vi "Day 9-2.vi"() -> ()   [LabVIEW 2020]
uses:
  Visit Item.ctl
panel:
  out "Answer":i32
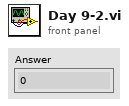
[diagram p1: front panel]
types:
  T1 = typedef "Visit Item.ctl" = cluster{"To":cluster{"Row":i32, "Col":i32}, "From":cluster{"Row":i32, "Col":i32}}
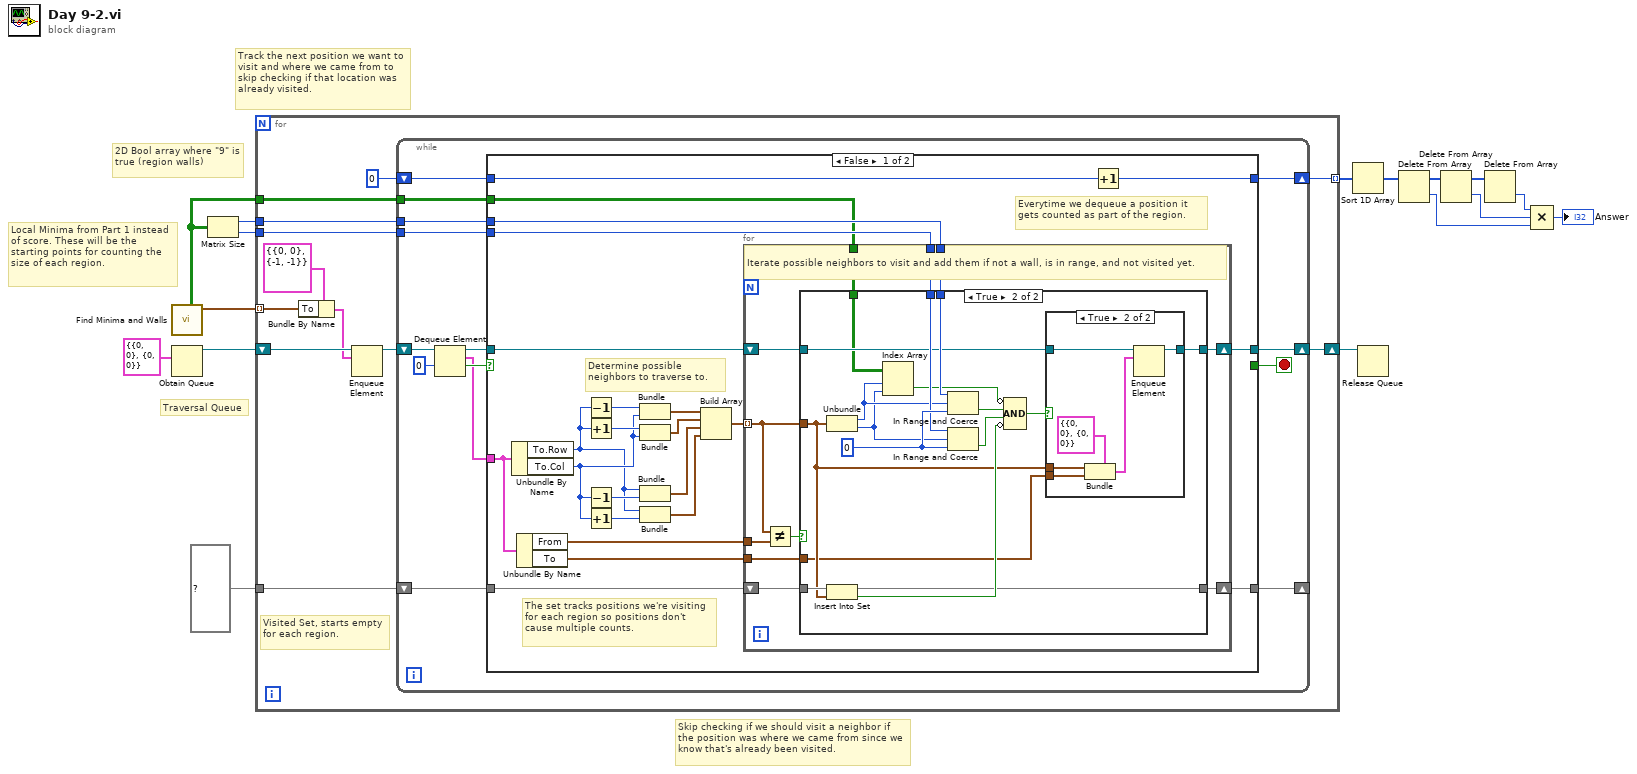
[diagram p0: block diagram]
diagram:
  # "Skip checking if we should visit a neighbor if the position was where we came from since we know that's already been visited."
  # "Track the next position we want to visit and where we came from to skip checking if that location was already visited."
  # "Local Minima from Part 1 instead of score. These will be the starting points for counting the size of each region."
  # "2D Bool array where \"9\" is true (region walls)"
  # "Traversal Queue"
  n1 = call "Find Minima and Walls.vi"() -> ("Low Points"=w16:cluster{i32, i32}[], "Wall"=w3:bool[][])  [unwired: 10 in]
  n2 = Obtain Queue(element data type=T1 {"To"={"Row"=0, "Col"=0}, "From"={"Row"=0, "Col"=0}} ("Visit Item")) -> (queue out=w14:refnum<queue>)  [unwired: 4 in, 2 out]
  n3 = Matrix Size(0:w3) -> (1:w2:i32, 2:w1:i32)
  n4 = for {
    tunnel: w16 -> [w27] mode=indexing
    shift-right: [w21] -> w12
    shift-left: w14 -> [w26]
    tunnel: w3 -> [w22]
    tunnel: set{cluster{"Row":i32, "Col":i32}} {} ("set") -> [w24]
    tunnel: [w19] -> w11 mode=indexing
    tunnel: w2 -> [w18]
    tunnel: w1 -> [w17]
    # "Visited Set, starts empty for each region."
    n5 = Bundle By Name(cluster=T1 {"To"={"Row"=0, "Col"=0}, "From"={"Row"=-1, "Col"=-1}} ("Visit Item"), "To"=w27) -> (w25:T1)
    n6 = Enqueue Element(queue=w26, element=w25) -> (queue out=w23:refnum<queue>)  [unwired: 2 in, 2 out]
    n7 = while {
      tunnel: w22 -> [w37]
      shift-right: [w31] -> _
      shift-left: w24 -> [w36]
      shift-right: [w34] -> w21
      shift-left: w23 -> [w42]
      shift-right: [w32] -> w19
      shift-left: 0 -> [w33]
      tunnel: w18 -> [w30]
      tunnel: w17 -> [w29]
      stop <- w35 stop-if-true
      n8 = Dequeue Element(queue=w42, timeout in ms (-1)=0) -> (queue out=w40:refnum<queue>, element=w38:T1, timed out?=w39:bool)  [unwired: 1 in, 1 out]
      n9 = case shown="False" w39 {
        selector: w39 -> [_ w106]
        tunnel: w40 -> [w52 w105]
        tunnel: w38 -> [w65 _]
        tunnel: w37 -> [w44 _]
        tunnel: w36 -> [w50 w103]
        tunnel: [_ w106] -> w35
        tunnel: [w51 w105] -> w34
        tunnel: w33 -> [w54 w104]
        tunnel: [w53 w104] -> w32
        tunnel: [w49 w103] -> w31
        tunnel: w30 -> [w47 _]
        tunnel: w29 -> [w46 _]
        frame False {
          # "The set tracks positions we're visiting for each region so positions don't cause multiple counts."
          # "Determine possible neighbors to traverse to."
          # "Everytime we dequeue a position it gets counted as part of the region."
          n10 = Unbundle By Name(w65) -> ("To.Row"=w59:i32, "To.Col"=w62:i32)
          n11 = Unbundle By Name(w65) -> ("From"=w45:cluster{"Row":i32, "Col":i32}, "To"=w43:cluster{"Row":i32, "Col":i32})
          n12 = Decrement(x=w59) -> (x-1=w64:i32)
          n13 = Increment(x=w59) -> (x+1=w63:i32)
          n14 = Decrement(x=w62) -> (x-1=w61:i32)
          n15 = Increment(x=w62) -> (x+1=w60:i32)
          n16 = Bundle(w64, "Col"=w62) -> (w58:cluster{i32, "Col":i32})  [unwired: 1 in]
          n17 = Bundle(w63, "Col"=w62) -> (w57:cluster{i32, "Col":i32})  [unwired: 1 in]
          n18 = Bundle("Row"=w59, w61) -> (w56:cluster{"Row":i32, i32})  [unwired: 1 in]
          n19 = Bundle("Row"=w59, w60) -> (w55:cluster{"Row":i32, i32})  [unwired: 1 in]
          n20 = Build Array(w58, w57, w56, w55) -> (w48:cluster{"Row":i32, "Col":i32}[])
          n21 = for {
            shift-right: [w67] -> w51
            shift-left: w52 -> [w70]
            shift-right: [w66] -> w49
            shift-left: w50 -> [w76]
            tunnel: w48 -> [w72] mode=indexing
            tunnel: w47 -> [w75]
            tunnel: w46 -> [w74]
            tunnel: w45 -> [w73]
            tunnel: w44 -> [w69]
            tunnel: w43 -> [w68]
            # "Iterate possible neighbors to visit and add them if not a wall, is in range, and not visited yet."
            n22 = Not Equal?(x=w72, y=w73) -> (x != y?=w71:bool)
            n23 = case shown="True" w71 {
              tunnel: w76 -> [w78 w95]
              tunnel: w75 -> [_ w93]
              tunnel: w74 -> [_ w92]
              tunnel: w72 -> [_ w83]
              tunnel: w70 -> [w77 w88]
              tunnel: w69 -> [_ w87]
              tunnel: w68 -> [_ w81]
              tunnel: [w77 w80] -> w67
              tunnel: [w78 w79] -> w66
              frame False {
              }
              frame True {
                w94 = 0 ("lower limit")
                n24 = Unbundle(w83) -> ("Row"=w86:i32, "Col"=w82:i32)
                n25 = Insert Into Set(10:w83, 11:w95) -> (2:w89:bool, 3:w79:set{cluster{"Row":i32, "Col":i32}})
                n26 = Index Array(array=w87, index (row)=w86, index (col)=w82) -> (element=w85:bool)
                n27 = In Range and Coerce(upper limit=w93, x=w86, lower limit=w94) -> (In Range?=w91:bool)  [unwired: 1 out]
                n28 = In Range and Coerce(upper limit=w92, x=w82, lower limit=w94) -> (In Range?=w90:bool)  [unwired: 1 out]
                n29 = Compound Arithmetic op=AND(invert w85, w91, w90, invert w89) -> (w84:bool)
                n30 = case shown="True" w84 {
                  tunnel: w88 -> [w96 w102]
                  tunnel: w83 -> [_ w101]
                  tunnel: w81 -> [_ w100]
                  tunnel: [w96 w98] -> w80
                  frame False {
                  }
                  frame True {
                    n31 = Bundle(cluster=T1 {"To"={"Row"=0, "Col"=0}, "From"={"Row"=0, "Col"=0}} ("Visit Item"), "To"=w101, "From"=w100) -> (w99:T1)
                    n32 = Enqueue Element(queue=w102, element=w99) -> (queue out=w98:refnum<queue>)  [unwired: 2 in, 2 out]
                  }
                }
              }
            }
          }
          n33 = Increment(x=w54) -> (x+1=w53:i32)
        }
        frame True {
          # "No more positions available for this region, it's done! Let the count fall out of the loop."
        }
      }
    }
  }
  n34 = Sort 1D Array(array=w11) -> (sorted array=w10:i32[])
  n35 = Release Queue(queue=w12) -> ()  [unwired: 2 in, 3 out]
  n36 = Delete From Array(array=w10) -> (deleted portion=w5:i32, array with subset deleted=w9:i32[])  [unwired: 2 in]
  n37 = Delete From Array(array=w9) -> (deleted portion=w6:i32, array with subset deleted=w8:i32[])  [unwired: 2 in]
  n38 = Delete From Array(array=w8) -> (deleted portion=w7:i32)  [unwired: 2 in, 1 out]
  n39 = Compound Arithmetic op=MULTIPLY(w7, w6, w5) -> (→"Answer":i32)
